vi "3.Digital Input - Polling a Button.vi"   [LabVIEW 2014]
doc: "This example shows how to read a digital input on an Arduino target, This example assumes a switch is wired to the digital input, therefore it implements debouncing when the input changes to a low state. A digital output is toggled when the switch is pressed."
uses:
  <vilib>/Aledyne-TSXperts/Arduino Compatible Compiler for LabVIEW/Code Generator/Arduino APIs/Digital/PinDirection.ctl
  <vilib>/Aledyne-TSXperts/Arduino Compatible Compiler for LabVIEW/Arduino Compatible Compiler for LabVIEW.lvlib
panel:
  # "Overview: Demonstrates how to read the state of a digital pin on an Arduino target.  An output pin is toggled when the input pin state changes.\n\nInstructions:\n1. Wire an LED's anode to a digital pin on the Arduino board and wire the cathode to a ground pin through a 220ohm or equivalent resistor (or use the onboard LED on pin 13).\n2. Wire one side of a button to a digital pin on the Arduino board and the other end to a ground pin.\n3. Set the Digital Pin wired below.\n4.  If this example has been loaded from the Arduino Compatible Compiler for LabVIEW, simply select Compile and Download.  Otherwise, open Tools>Arduino Compatible Compiler for LabVIEW in LabVIEW, then select File>Load VI, and select this VI and then Compile and Download.\n5. Observe the LED turning off and on when the switch is pressed."
types:
  T1 = typedef "Arduino Compatible Compiler for LabVIEW.lvlib/PinDirection.ctl" = enum16{" INPUT", "OUTPUT", " INPUT_PULLUP"}
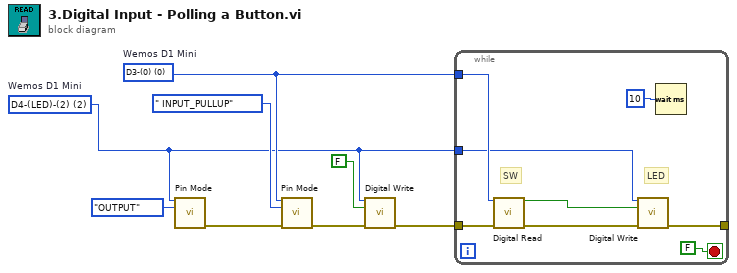
[diagram p0: block diagram]
diagram:
  w1 = u8 2 items=["D0-(16)"=16, "D1-SCL(5)"=5, "D2-SDA(4)"=4, "D3-(0)"=0, "D4-(LED)-(2)"=2, "D5-SCK(14)"=14, "D6-MISO(12)"=12, "D7-MOSI(13)"=13, "D8-SS(15)"=15, "TX(3)"=3, "RX(1)"=1, "ADC0,(17)"=17]  # Wemos D1 Mini
  w2 = u8 0 items=["D0-(16)"=16, "D1-SCL(5)"=5, "D2-SDA(4)"=4, "D3-(0)"=0, "D4-(LED)-(2)"=2, "D5-SCK(14)"=14, "D6-MISO(12)"=12, "D7-MOSI(13)"=13, "D8-SS(15)"=15, "TX(3)"=3, "RX(1)"=1, "ADC0,(17)"=17]  # Wemos D1 Mini
  n1 = call <vilib>:"Pin Mode.vi"("pin"=w1, "direction"=PinDirection."OUTPUT" ("Direction")) -> ("error out"=w6:errorcluster)  [unwired: 13 in]
  n2 = call <vilib>:"Pin Mode.vi"("pin"=w2, "direction"=PinDirection." INPUT_PULLUP" ("Direction"), "error in (no error)"=w6) -> ("error out"=w5:errorcluster)  [unwired: 12 in]
  n3 = call <vilib>:"Digital Write.vi"("pin"=w1, "state"=FALSE, "error in (no error)"=w5) -> ("error out"=w4:errorcluster)  [unwired: 12 in]
  n4 = while {
    tunnel: w1 -> [w12]
    tunnel: w4 -> [w15]
    tunnel: w2 -> [w13]
    tunnel: [w10] -> _
    stop <- FALSE stop-if-true
    # "SW"
    # "LED"
    n5 = call <vilib>:"Digital Read.vi"("pin"=w13, "error in (no error)"=w15) -> ("state"=w9:bool, "error out"=w11:errorcluster)  [unwired: 12 in]
    n6 = call <vilib>:"Digital Write.vi"("pin"=w12, "state"=w9, "error in (no error)"=w11) -> ("error out"=w10:errorcluster)  [unwired: 12 in]
    n7 = Wait (ms)(milliseconds to wait=u32 10) -> ()  [unwired: 1 out]
  }
